vi "handler_calibration.vi"(8 "error in (no error)":errorcluster, 11 "HTTP Request in":T1) -> (0 "error out":errorcluster, 1 "Handler name":string, 3 "HTTP Request out":T1)   [LabVIEW 2011]
uses:
  template_field_type.ctl
  http_field.ctl
  http_request.ctl
  http_response.ctl
  template_field.ctl
  http_request_response.ctl
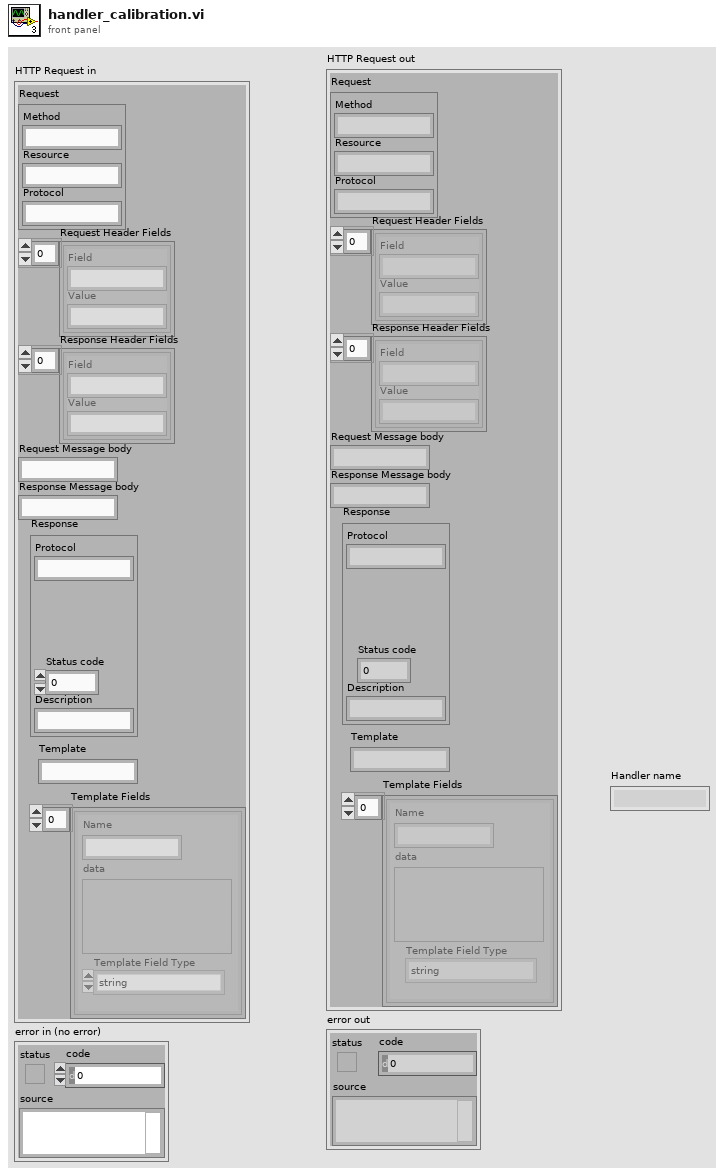
[diagram p1: front panel]
types:
  T1 = typedef "http_request_response.ctl" = cluster{"Request":T2, "Request Header Fields":T3[], "Response Header Fields":T3[], "Request Message body":string, "Response Message body":string, "Response":T4, "Template":string, "Template Fields":T5[]}
  T2 = typedef "http_request.ctl" = cluster{"Method":string, "Resource":string, "Protocol":string}
  T3 = typedef "http_field.ctl" = cluster{"Field":string, "Value":string}
  T4 = typedef "http_response.ctl" = cluster{"Protocol":string, "Status code":dbl, "Description":string}
  T5 = typedef "template_field.ctl" = cluster{"Name":string, "Template Field Type":T6, "data":variant}
  T6 = typedef "template_field_type.ctl" = enum16{"string", "string array", "number", "number array", "cluster", "cluster array"}
  T7 = typedef "html_form_field.ctl" = cluster{"field name":string, "field value":string}
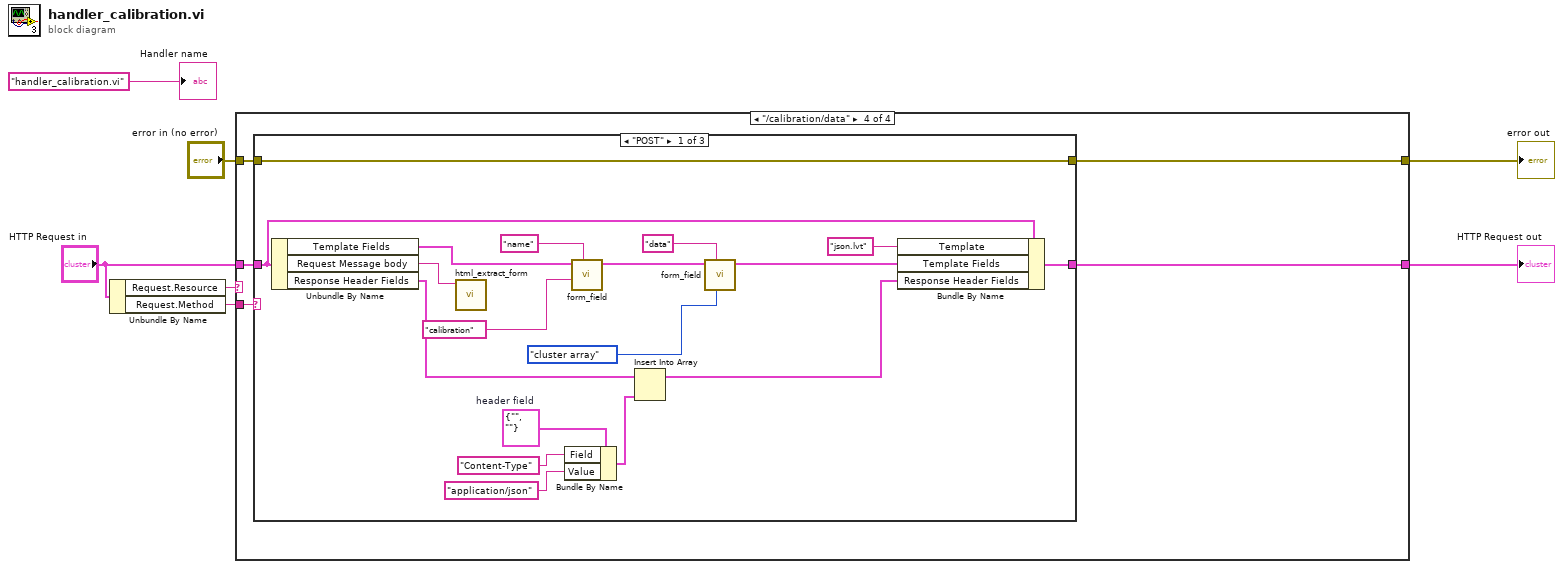
[diagram p0: block diagram]
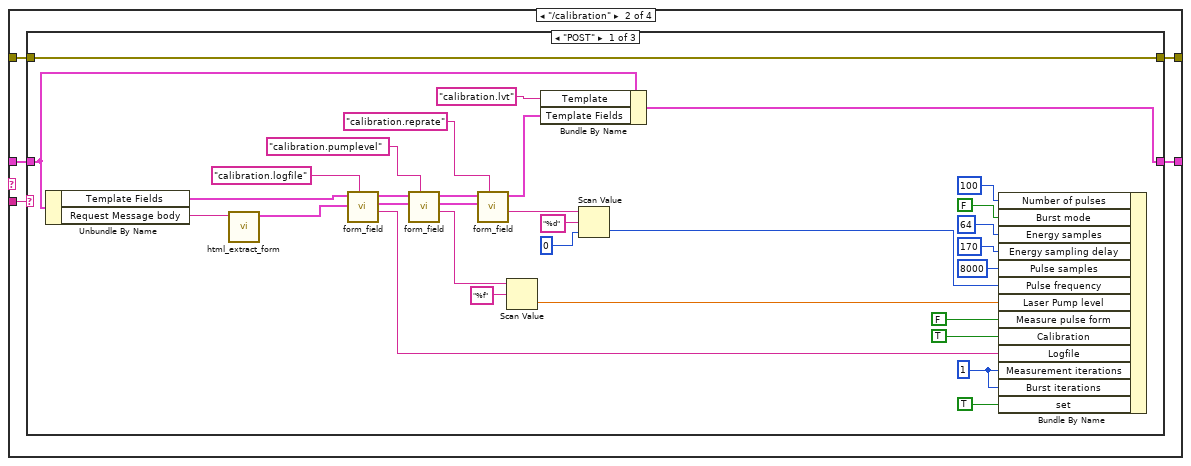
[diagram p3: hidden frame]
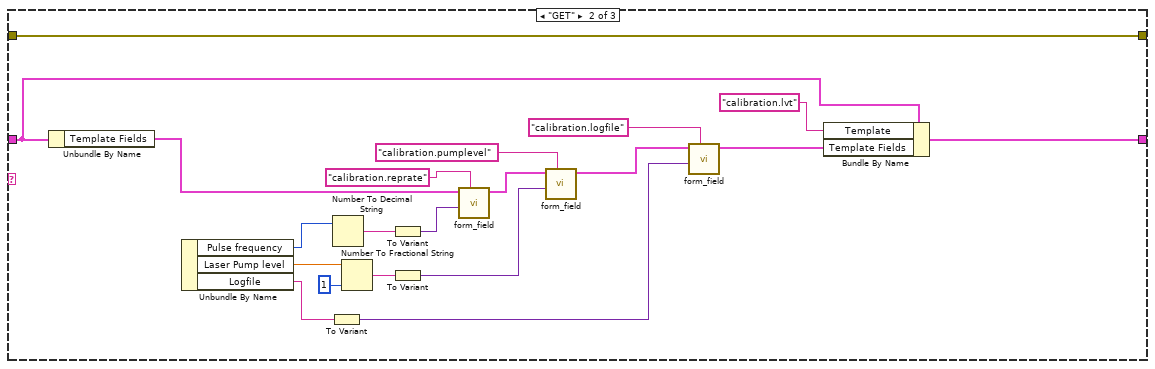
[diagram p4: hidden frame]
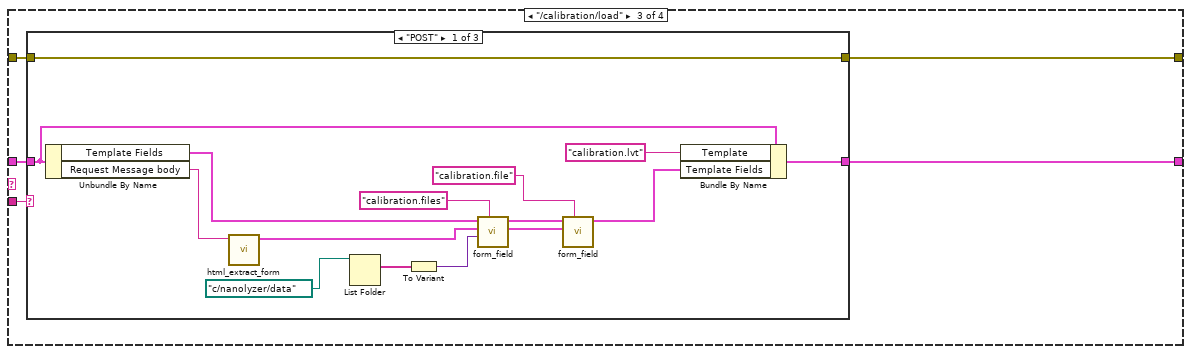
[diagram p6: hidden frame]
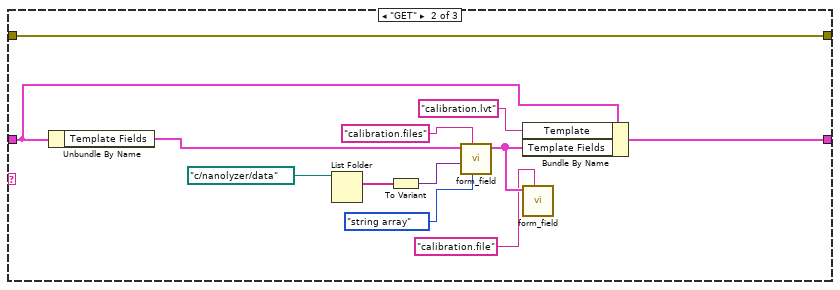
[diagram p7: hidden frame]
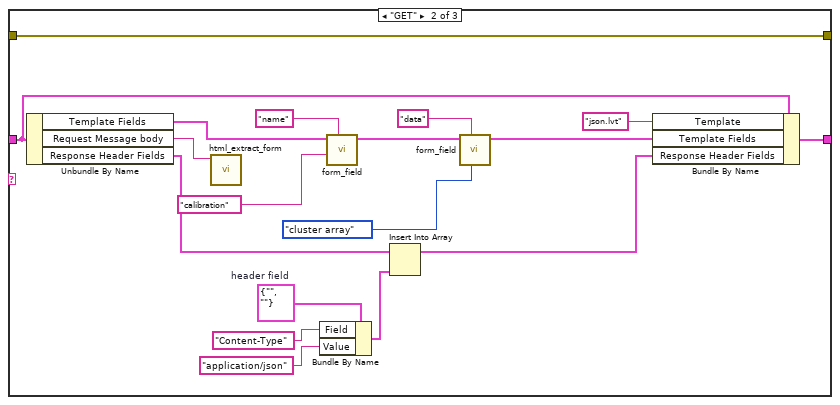
[diagram p9: hidden frame]
diagram:
  n1 = Unbundle By Name("HTTP Request in") -> ("Request.Resource"=w3:string, "Request.Method"=w2:string)
  n2 = case shown="\"/calibration/data\"" w3 {
    tunnel: w2 -> [_ w14 w73 w107]
    tunnel: "HTTP Request in" -> [w9 w13 w72 w106]
    tunnel: [w9 w12 w71 w105] -> w6
    tunnel: "error in (no error)" -> [w8 w11 w70 w104]
    tunnel: [w8 w10 w69 w103] -> w5
    frame Default {
    }
    frame "/calibration" {
      n3 = case shown="\"POST\"" w14 {
        tunnel: w13 -> [w44 w63 w68]
        tunnel: [w45 w65 w68] -> w12
        tunnel: w11 -> [w46 w66 w67]
        tunnel: [w46 w66 w67] -> w10
        frame "POST" {
          w29 = u32 1 ("Measurement iterations")
          n4 = Unbundle By Name(w44) -> ("Template Fields"=w27:T5[], "Request Message body"=w43:string)
          n5 = call "html_extract_form.vi"("Message Body"=w43) -> ("Form Data"=w22:T7[])  [unwired: 10 in]
          n6 = call "form_field.vi"("Name"="calibration.logfile", "Form Data"=w22, "Template Fields"=w27) -> ("field value"=w19:string, "Form Data"=w26:T7[], "Template Fields"=w23:T5[])  [unwired: 6 in]
          n7 = call "form_field.vi"("Name"="calibration.pumplevel", "Form Data"=w26, "Template Fields"=w23) -> ("field value"=w17:string, "Form Data"=w25:T7[], "Template Fields"=w24:T5[])  [unwired: 6 in]
          n8 = call "form_field.vi"("Name"="calibration.reprate", "Form Data"=w25, "Template Fields"=w24) -> ("field value"=w15:string, "Template Fields"=w21:T5[])  [unwired: 6 in, 1 out]
          n9 = Scan Value(string=w17, format string="%f") -> (value=w37:dbl)  [unwired: 1 in, 1 out]
          n10 = Bundle By Name(cluster=w44, "Template"="calibration.lvt", "Template Fields"=w21) -> (w45:T1)
          n11 = Scan Value(string=w15, format string="%d", default (0 dbl)=u32 0) -> (value=w39:u32)  [unwired: 1 out]
          n12 = Bundle By Name("Number of pulses"=u16 100, "Burst mode"=FALSE, "Energy samples"=u16 64, "Energy sampling delay"=u32 170, "Pulse samples"=u16 8000, "Pulse frequency"=w39, "Laser Pump level"=w37, "Measure pulse form"=FALSE, "Calibration"=TRUE, "Logfile"=w19, "Measurement iterations"=w29, "Burst iterations"=w29, "set"=TRUE) -> ()  [unwired: 1 in, 1 out]
        }
        frame "GET" {
          n13 = Unbundle By Name(w63) -> ("Template Fields"=w56:T5[])
          n14 = Unbundle By Name() -> ("Pulse frequency"=w61:u16, "Laser Pump level"=w60:dbl, "Logfile"=w58:string)  [unwired: 1 in]
          n15 = To Variant(anything=w58) -> (Variant=w50:variant)
          n16 = Number To Decimal String(number=w61) -> (decimal integer string=w62:string)  [unwired: 1 in]
          n17 = Number To Fractional String(number=w60, precision (6)=i16 1) -> (F-format string=w59:string)  [unwired: 2 in]
          n18 = To Variant(anything=w62) -> (Variant=w52:variant)
          n19 = To Variant(anything=w59) -> (Variant=w51:variant)
          n20 = call "form_field.vi"("Name"="calibration.reprate", "Value"=w52, "Template Fields"=w56) -> ("Template Fields"=w55:T5[])  [unwired: 6 in, 2 out]
          n21 = call "form_field.vi"("Name"="calibration.pumplevel", "Value"=w51, "Template Fields"=w55) -> ("Template Fields"=w54:T5[])  [unwired: 6 in, 2 out]
          n22 = call "form_field.vi"("Name"="calibration.logfile", "Value"=w50, "Template Fields"=w54) -> ("Template Fields"=w53:T5[])  [unwired: 6 in, 2 out]
          n23 = Bundle By Name(cluster=w63, "Template"="calibration.lvt", "Template Fields"=w53) -> (w65:T1)
        }
        frame Default {
        }
      }
    }
    frame "/calibration/load" {
      n24 = case shown="\"POST\"" w73 {
        tunnel: w72 -> [w86 w97 w102]
        tunnel: [w87 w99 w102] -> w71
        tunnel: w70 -> [w88 w100 w101]
        tunnel: [w88 w100 w101] -> w69
        frame "POST" {
          n25 = Unbundle By Name(w86) -> ("Template Fields"=w83:T5[], "Request Message body"=w85:string)
          n26 = call "html_extract_form.vi"("Message Body"=w85) -> ("Form Data"=w82:T7[])  [unwired: 10 in]
          n27 = List Folder(path=path "c:/nanolyzer/data") -> (filenames=w75:string[])  [unwired: 3 in, 3 out]
          n28 = To Variant(anything=w75) -> (Variant=w74:variant)
          n29 = call "form_field.vi"("Name"="calibration.files", "Value"=w74, "Form Data"=w82, "Template Fields"=w83) -> ("Form Data"=w79:T7[], "Template Fields"=w80:T5[])  [unwired: 5 in, 1 out]
          n30 = call "form_field.vi"("Name"="calibration.file", "Form Data"=w79, "Template Fields"=w80) -> ("Template Fields"=w78:T5[])  [unwired: 6 in, 2 out]
          n31 = Bundle By Name(cluster=w86, "Template"="calibration.lvt", "Template Fields"=w78) -> (w87:T1)
        }
        frame "GET" {
          n32 = Unbundle By Name(w97) -> ("Template Fields"=w96:T5[])
          n33 = List Folder(path=path "c:/nanolyzer/data") -> (filenames=w91:string[])  [unwired: 3 in, 3 out]
          n34 = To Variant(anything=w91) -> (Variant=w95:variant)
          n35 = call "form_field.vi"("Template Field Type"=template_field_type."string array", "Name"="calibration.files", "Value"=w95, "Template Fields"=w96) -> ("Template Fields"=w90:T5[])  [unwired: 5 in, 2 out]
          n36 = Bundle By Name(cluster=w97, "Template"="calibration.lvt", "Template Fields"=w90) -> (w99:T1)
          n37 = call "form_field.vi"("Name"="calibration.file", "Template Fields"=w90) -> ()  [unwired: 7 in, 3 out]
        }
        frame Default {
        }
      }
    }
    frame "/calibration/data" {
      n38 = case shown="\"POST\"" w107 {
        tunnel: w106 -> [w123 w141 w145]
        tunnel: [w124 w142 w145] -> w105
        tunnel: w104 -> [w125 w143 w144]
        tunnel: [w125 w143 w144] -> w103
        frame "POST" {
          w112 = T3 {"Field"="", "Value"=""}  # header field
          n39 = Unbundle By Name(w123) -> ("Template Fields"=w118:T5[], "Request Message body"=w122:string, "Response Header Fields"=w113:T3[])
          n40 = call "html_extract_form.vi"("Message Body"=w122) -> ()  [unwired: 10 in, 1 out]
          n41 = Bundle By Name(cluster=w112, "Field"="Content-Type", "Value"="application/json") -> (w111:T3)
          n42 = call "form_field.vi"("Name"="name", "Value"="calibration" ("Name"), "Template Fields"=w118) -> ("Template Fields"=w115:T5[])  [unwired: 6 in, 2 out]
          n43 = Insert Into Array(array=w113, new element=w111) -> (w114:T3[])  [unwired: 1 in]
          n44 = call "form_field.vi"("Template Field Type"=template_field_type."cluster array", "Name"="data", "Template Fields"=w115) -> ("Template Fields"=w108:T5[])  [unwired: 6 in, 2 out]
          n45 = Bundle By Name(cluster=w123, "Template"="json.lvt", "Template Fields"=w108, "Response Header Fields"=w114) -> (w124:T1)
        }
        frame "GET" {
          w131 = T3 {"Field"="", "Value"=""}  # header field
          n46 = Unbundle By Name(w141) -> ("Template Fields"=w136:T5[], "Request Message body"=w140:string, "Response Header Fields"=w132:T3[])
          n47 = call "html_extract_form.vi"("Message Body"=w140) -> ()  [unwired: 10 in, 1 out]
          n48 = Bundle By Name(cluster=w131, "Field"="Content-Type", "Value"="application/json") -> (w130:T3)
          n49 = call "form_field.vi"("Name"="name", "Value"="calibration" ("Name"), "Template Fields"=w136) -> ("Template Fields"=w127:T5[])  [unwired: 6 in, 2 out]
          n50 = Insert Into Array(array=w132, new element=w130) -> (w133:T3[])  [unwired: 1 in]
          n51 = call "form_field.vi"("Template Field Type"=template_field_type."cluster array", "Name"="data", "Template Fields"=w127) -> ("Template Fields"=w126:T5[])  [unwired: 6 in, 2 out]
          n52 = Bundle By Name(cluster=w141, "Template"="json.lvt", "Template Fields"=w126, "Response Header Fields"=w133) -> (w142:T1)
        }
        frame Default {
        }
      }
    }
  }
  "HTTP Request out" <- w6
  "error out" <- w5
  "Handler name" <- "handler_calibration.vi" ("Handler name")
